vi "Add Frames.vi"(8 "error in (no error)":errorcluster, 9 "Frames":T3[](array[typedef]), 10 "Action":T2, 11 "Section Ref in":T1 format="%.0x") -> (0 "error out":errorcluster, 3 "Section Ref out":T1 format="%.0x")   [LabVIEW 2015, in "J1939 System Definition API Support.lvlib"]
uses:
  J1939 System Definition API Support.lvlib
  Types/Add Item - Frame Cluster.ctl
  Types/Remove Frame Action.ctl
  <vilib>/NI Veristand/Custom Device API/Custom Device Item Ref.ctl
  Shared/SubVIs/Constants.vi
  <vilib>/NI/NIVS System Definition Utilities/_SubVIs/SysDef.Search.GUID.vi
  Shared/J1939 Addon Shared.lvlib
  <vilib>/NI/NIVS System Definition Utilities/System Definition Utilities.lvlib
  <vilib>/NI VeriStand/Custom Device API/Custom Device API.lvlib
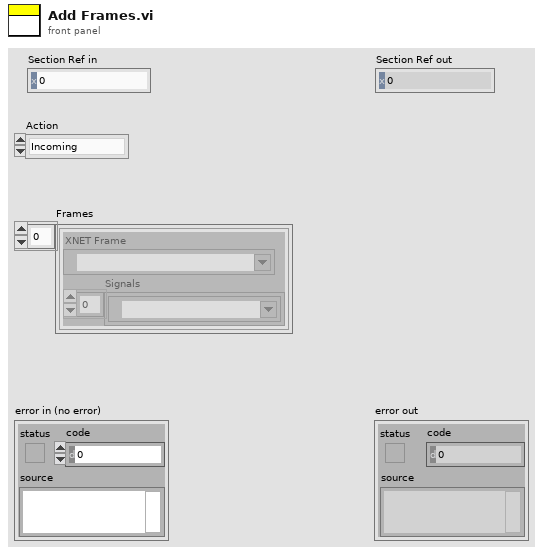
[diagram p1: front panel]
types:
  T1 = typedef "Custom Device API.lvlib/Custom Device Item Ref.ctl" = u64
  T2 = typedef "J1939 System Definition API Support.lvlib/Remove Frame Action.ctl" = enum16{"Incoming", "Outgoing Event", "Outgoing Cyclic"}
  T3 = typedef "J1939 System Definition API Support.lvlib/Add Item - Frame Cluster.ctl" = cluster{"XNET Frame":refnum<k21>, "Signals":refnum<k21>[]}
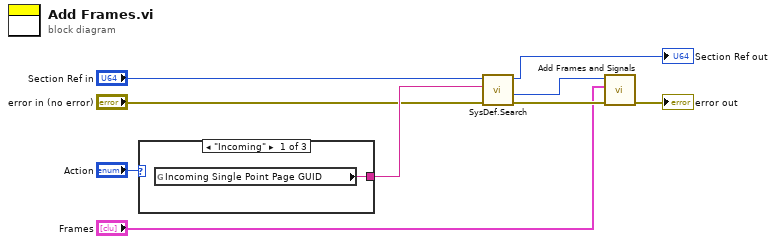
[diagram p0: block diagram]
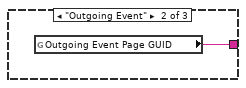
[diagram p2: hidden frame]
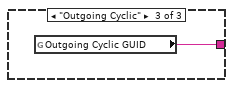
[diagram p3: hidden frame]
diagram:
  n1 = case shown="\"Incoming\"" "Action" {
    tunnel: [w10 w11 w12] -> w4
    frame "Incoming" {
      n2 = global read "Constants.vi" "Incoming Single Point Page GUID"() -> (w10:string)
    }
    frame "Outgoing Event" {
      n3 = global read "Constants.vi" "Outgoing Event Page GUID"() -> (w11:string)
    }
    frame "Outgoing Cyclic" {
      n4 = global read "Constants.vi" "Outgoing Cyclic GUID"() -> (w12:string)
    }
  }
  n5 = call-poly <vilib>:"SysDef.Search.vi"("error in (no error)"="error in (no error)", "GUID"=w4, "nodeID"="Section Ref in") -> ("error out"=w9:errorcluster, "Value out"=w8:u64, "nodeID out"=→"Section Ref out":u64)  [unwired: 5 in, 1 out]
  n6 = call "Add Frames and Signals.vi"("error in"=w9, "Frames"="Frames", "Parent Ref in"=w8) -> ("error out"=→"error out":errorcluster)  [unwired: 7 in, 1 out]
